vi "Begin.vi"() -> (1 "CameraDevRef":T5)   [LabVIEW 2011]
doc: "Called before other user functions, this VI is expected to open initial I/O refnums, load in file data, and do all program initialization. Notice that the <B>error out</B> terminal is simply used for data flow. Wiring it to other structures or subVIs ensures that this VI runs first."
uses:
  <vilib>/Rock Robotics/WPI/Camera/WPI_CameraDevRef.ctl
  <vilib>/Rock Robotics/WPI/Encoder/WPI_EncoderDevRef.ctl
  <vilib>/Rock Robotics/SystemInterfaces/Encoder/FPGA_EncoderIdx.ctl
  <vilib>/Rock Robotics/SystemInterfaces/Counter/FPGA_CounterCtrSystemIndex.ctl
  <vilib>/Rock Robotics/WPI/Encoder/WPI_EncoderType.ctl
  <vilib>/Rock Robotics/WPI/Joystick/WPI_JoystickDeviceEnum.ctl
  <vilib>/Rock Robotics/SystemInterfaces/DIO/FPGA_DIOPWMChannel.ctl
  <vilib>/Rock Robotics/SystemInterfaces/Typedef/FPGA_TypedefDigitalModule.ctl
  <vilib>/Rock Robotics/WPI/MotorControl/WPI_MotorControlOpen Victor.vi
  Robot Global Data.vi
  <vilib>/Rock Robotics/SystemInterfaces/DIO/FPGA_DIORelayChannel.ctl
  <vilib>/Rock Robotics/WPI/Relay/WPI_RelayDirection.ctl
  <vilib>/Rock Robotics/SystemInterfaces/AI/FPGA_AIChannel.ctl
  <vilib>/Rock Robotics/WPI/Counter/WPI_CounterDigitalInputToDigitalSource.vi
  <vilib>/Rock Robotics/SystemInterfaces/DIO/FPGA_DIOChannel.ctl
  <vilib>/Rock Robotics/SystemInterfaces/AI/FPGA_AIGyroChannel.ctl
  <vilib>/Rock Robotics/WPI/MotorControl/WPI_MotorControlOpen Jaguar.vi
  <vilib>/Rock Robotics/SystemInterfaces/Typedef/FPGA_TypedefAnalogModule.ctl
  <vilib>/Utility/file.llb/Read From Spreadsheet File (DBL).vi
panel:
  out "source":string
  out "code":i32
  out "LDriveEncoder 3":cluster{"status":bool}
  out "EncoderDevRef 3":T1={"DevStatus"={"status"=FALSE, "code"=0, "source"=""}, "EncoderIndex"=enum."Invalid", "CounterIndex"=enum."Invalid", "DistancePerCount"=1.0, "Decoding Type"=enum."4x"}
  out "EncoderDevRef 2":T1={"DevStatus"={"status"=FALSE, "code"=0, "source"=""}, "EncoderIndex"=enum."Invalid", "CounterIndex"=enum."Invalid", "DistancePerCount"=1.0, "Decoding Type"=enum."4x"}
  out "LDriveEncoder 2":errorcluster
  out "EncoderDevRef":T1={"DevStatus"={"status"=FALSE, "code"=0, "source"=""}, "EncoderIndex"=enum."Invalid", "CounterIndex"=enum."Invalid", "DistancePerCount"=1.0, "Decoding Type"=enum."4x"}
  out "LDriveEncoder":errorcluster
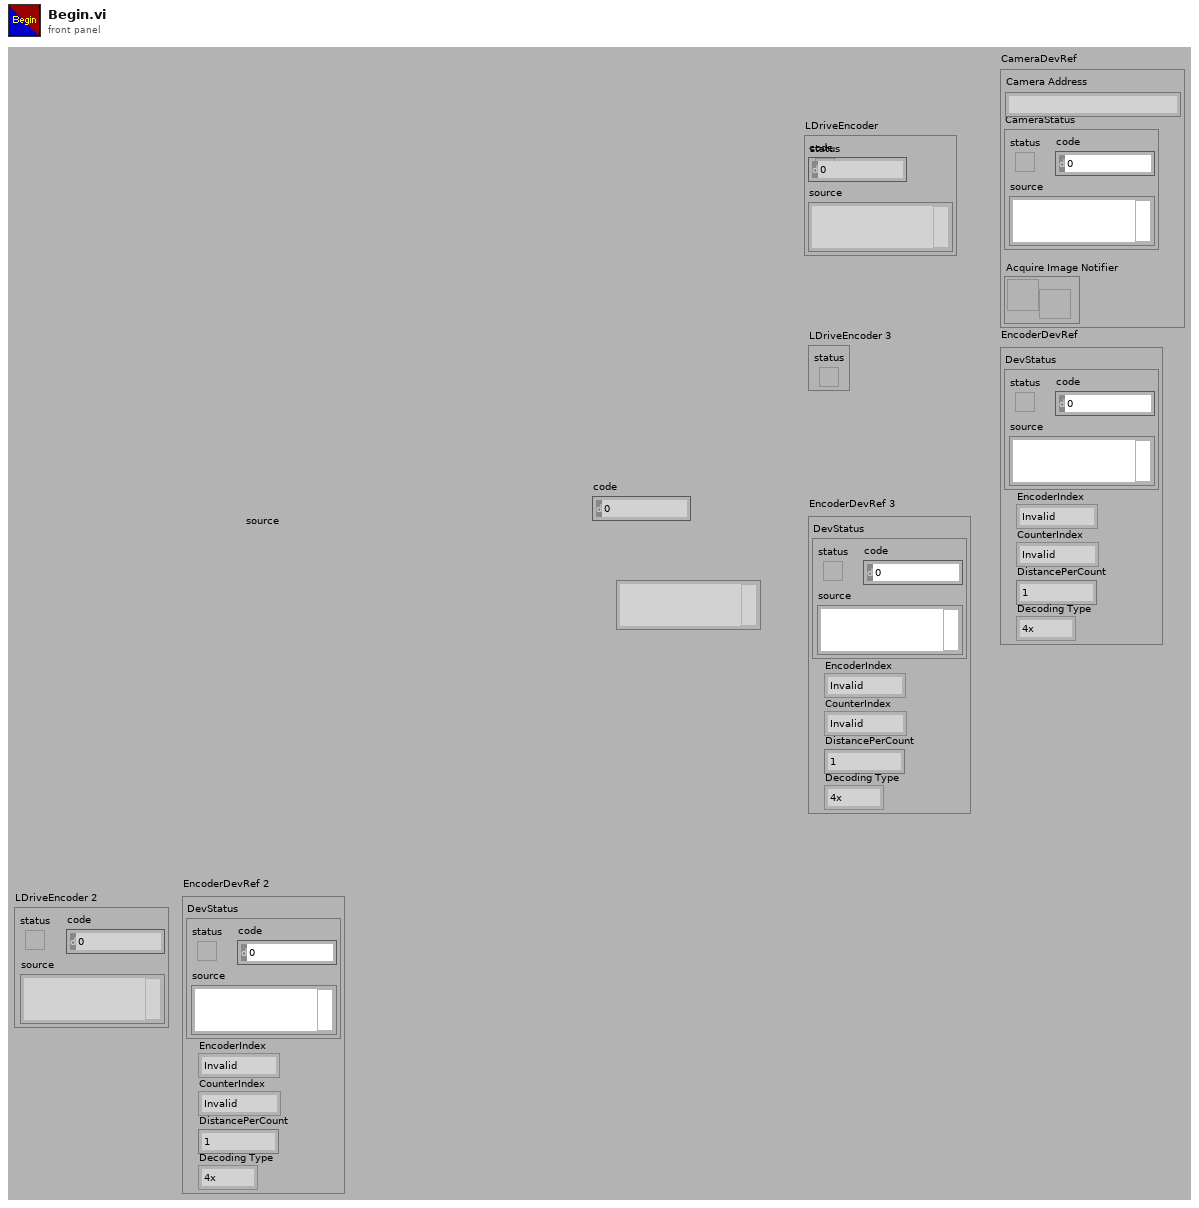
[diagram p1: front panel]
types:
  T1 = typedef "WPI_EncoderDevRef.ctl" = cluster{"DevStatus":errorcluster, "EncoderIndex":T2, "CounterIndex":T3, "DistancePerCount":dbl, "Decoding Type":T4}
  T2 = typedef "FPGA_EncoderIdx.ctl" = enum8{"Enc 0", "Enc 1", "Enc 2", "Enc 3", "Invalid"}
  T3 = typedef "FPGA_CounterCtrSystemIndex.ctl" = enum8{"Ctr 0", "Ctr 1", "Ctr 2", "Ctr 3", "Ctr 4", "Ctr 5", "Ctr 6", "Ctr 7", "Invalid"}
  T4 = typedef "WPI_EncoderType.ctl" = enum16{"1x", "2x", "4x"}
  T5 = typedef "WPI_CameraDevRef.ctl" = cluster{"Camera Address":string, "CameraStatus":errorcluster, "Acquire Image Notifier":refnum<notifier>}
  T6 = typedef "FPGA_TypedefDigitalModule.ctl" = enum16{"Digital Module 1", "Digital Module 2"}
  T7 = typedef "FPGA_DIOPWMChannel.ctl" = enum8{"PWM 1", "PWM 2", "PWM 3", "PWM 4", "PWM 5", "PWM 6", "PWM 7", "PWM 8", "PWM 9", "PWM 10", "Invalid"}
  T8 = typedef "WPI_JoystickDeviceEnum.ctl" = enum16{"USB 1", "USB 2", "USB 3", "USB 4", "Kinect 1", "Kinect 2"}
  T9 = typedef "FPGA_DIORelayChannel.ctl" = enum8{"Relay 1", "Relay 2", "Relay 3", "Relay 4", "Relay 5", "Relay 6", "Relay 7", "Relay 8", "Invalid"}
  T10 = typedef "FPGA_DIOChannel.ctl" = enum8{"DIO 1", "DIO 2", "DIO 3", "DIO 4", "DIO 5", "DIO 6", "DIO 7", "DIO 8", "DIO 9", "DIO 10", "DIO 11", "DIO 12", "DIO 13", "DIO 14", "Invalid"}
  T11 = typedef "WPI_MotorControlDeviceRef.ctl" = cluster{"DeviceStatus":errorcluster, "Type":enum16{"PWM", "CAN"}, "PWM":cluster{"Digital Module":T6, "PWM Channel":T7, "DeadBand":T12}, "CAN":cluster{"Device Number":u8, "Control Mode":T13, "Semaphore":T14, "Max Vout":dbl}, "Invert":bool, "TransformRef":T15, "InvTransformRef":T15}
  T12 = typedef "WPI_PWMDeadband.ctl" = cluster{"Name":string, "maxPositivePwm":i32, "minPositivePwm":i32, "centerPwm":i32, "maxNegativePwm":i32, "minNegativePwm":i32, "angularRange":u16}
  T13 = typedef "WPI_CANJaguar_ControlMode.ctl" = enum8{"Percent VBus", "Current", "Speed", "Position", "Voltage"}
  T14 = typedef "Semaphore RefNum" = refnum<k1>
  T15 = typedef "WPI_PWMTransform_ConPane.ctl" = refnum<vi>
  T16 = typedef "WPI_DigitalInputDevRef.ctl" = cluster{"DevStatus":errorcluster, "DIO Channel":T10, "Digital Module":T6}
  T17 = typedef "FPGA_CounterEncoderSourceConvertionLVSourceType.ctl" = cluster{"DevStatus":errorcluster, "AnalogTriggerMode?":bool, "DigitalMode":cluster{"Digital Module":T6, "DIO Channel":T18}, "AnalogTriggerMode":cluster{"AnalogTriggerIndex":T19, "OutputType":T20}}
  T18 = typedef "FPGA_DIODigitalSourceChannel.ctl" = enum8{"DIO 1", "DIO 2", "DIO 3", "DIO 4", "DIO 5", "DIO 6", "DIO 7", "DIO 8", "DIO 9", "DIO 10", "DIO 11", "DIO 12", "DIO 13", "DIO 14", "Disabled"}
  T19 = typedef "FPGA_AnalogTriggerIndex.ctl" = enum8{"Trig 0", "Trig 1", "Trig 2", "Trig 3", "Trig 4", "Trig 5", "Trig 6", "Trig 7", "Invalid"}
  T20 = typedef "FPGA_AnalogTriggerOutType.ctl" = enum16{"InWindow", "TriggerState", "Rising", "Falling"}
  T21 = typedef "WPI_RelayDevRef.ctl" = cluster{"DevStatus":errorcluster, "Relay Channel":T9, "Digital Module":T6, "Relay Direction":T22}
  T22 = typedef "WPI_RelayDirection.ctl" = enum16{"Both directions", "Forward only", "Reverse only"}
  T23 = typedef "FPGA_AIChannel.ctl" = enum8{"AI 1", "AI 2", "AI 3", "AI 4", "AI 5", "AI 6", "AI 7", "AI 8", "Invalid"}
  T24 = typedef "WPI_JoystickDevRef.ctl" = cluster{"Device":T8}
  T25 = typedef "WPI_AnalogChannelDevRef.ctl" = cluster{"DevStatus":errorcluster, "Analog Module":T26, "Analog Channel":T23}
  T26 = typedef "FPGA_TypedefAnalogModule.ctl" = enum16{"Analog Module 1", "Analog Module 2"}
  T27 = typedef "WPI_CameraImageSize.ctl" = enum16{"640x480", "320x240", "160x120"}
  T28 = cluster{"fps":i32, "compression":i32, "Image Size":T27}
  T29 = typedef "WPI_CameraWhite Balance Values.ctl" = enum16{"Auto", "Fixed indoor", "Fixed outdoor 1", "Fixed outdoor 2", "Fixed fluorescent 1", "Fixed fluorescent 2", "Hold current"}
  T30 = typedef "WPI_CameraExposure Values.ctl" = enum16{"Auto", "Flicker-free 50 Hz", "Flicker-free 60 Hz", "Hold current"}
  T31 = typedef "WPI_ServoDeviceRef.ctl" = cluster{"DeviceStatus":errorcluster, "Digital Module":T6, "PWM Channel":T7, "DeadBand":T12}
  T32 = typedef "FPGA_AIGyroChannel.ctl" = enum8{"AI 1", "AI 2", "Invalid"}
  T33 = typedef "WPI_GyroDevRef.ctl" = cluster{"DevStatus":errorcluster, "Analog Module":T26, "Analog Channel":T23, "Offset":dbl, "Gain (VoltsPerDegree/Second)":dbl}
  T34 = typedef "WPI_UltrasonicDeviceRef.ctl" = cluster{"DevStatus":errorcluster, "Ping Digital Module":T6, "Echo Digital Module":T6, "Ping Channel":T10, "Echo Channel":T10, "CntIndex":T3}
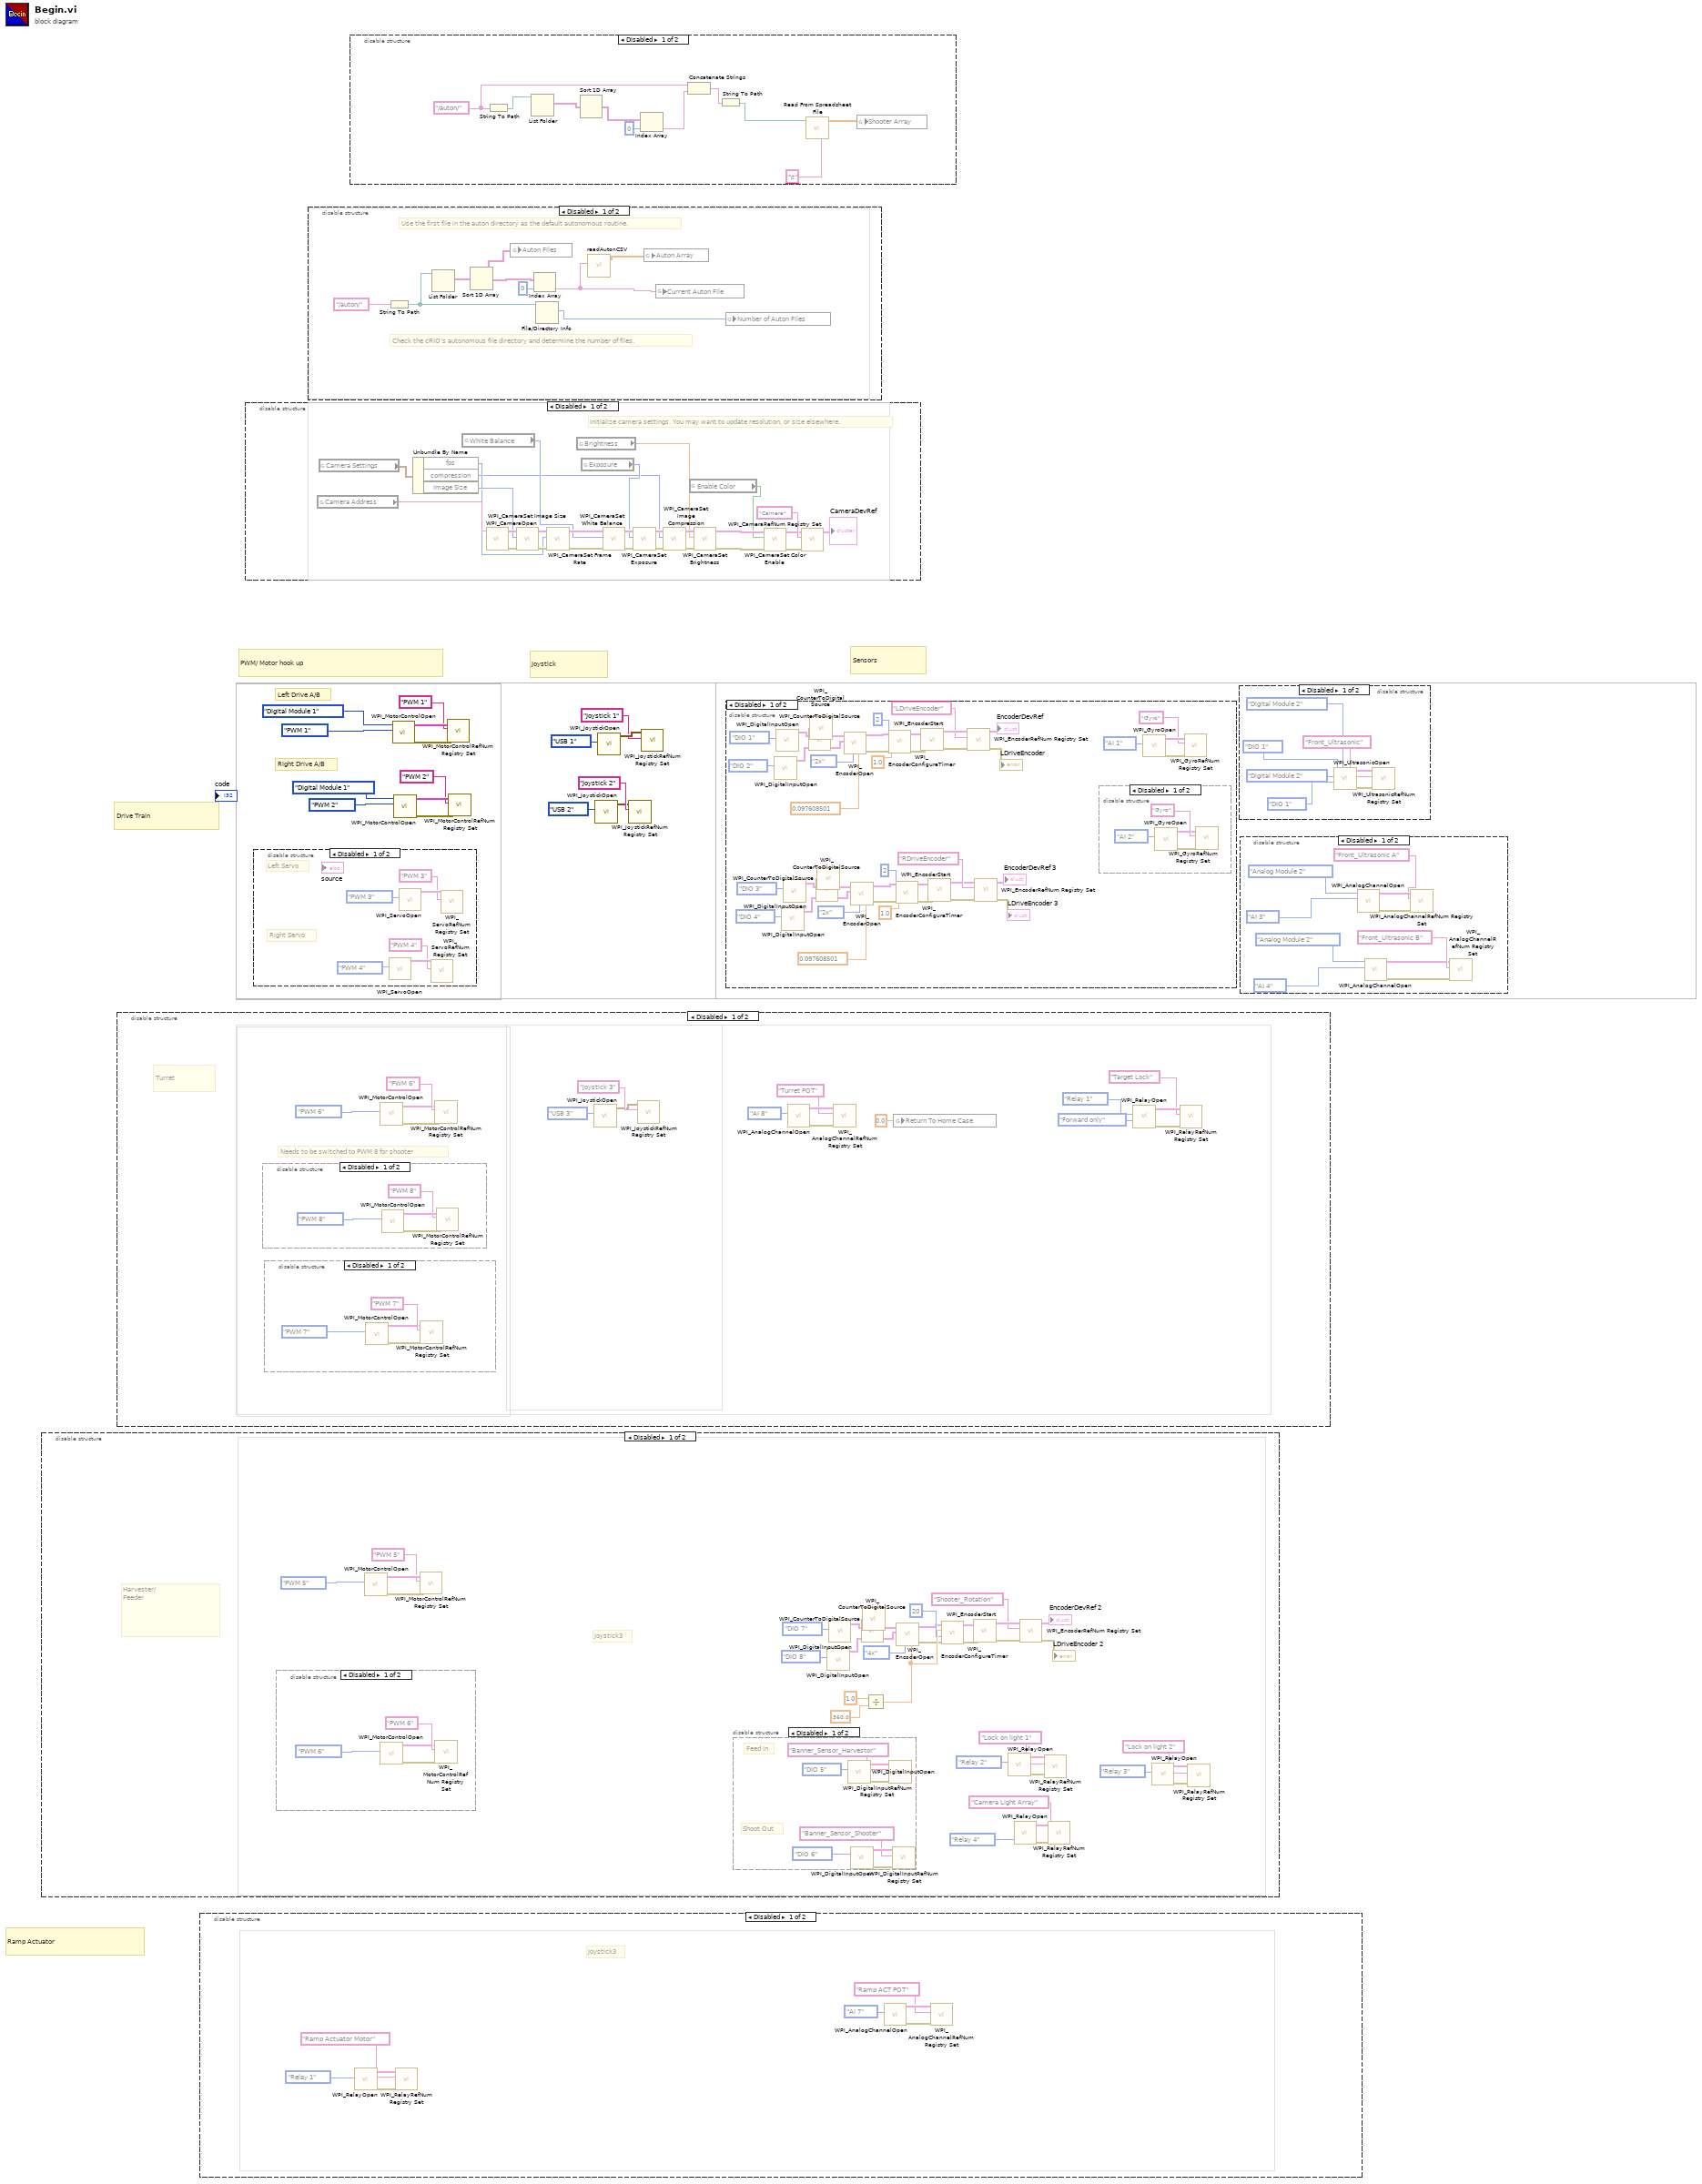
[diagram p0: block diagram]
diagram:
  # "Right Drive A/B"
  # "Left Drive A/B"
  # "Ramp Actuator"
  # "Drive Train"
  # "Sensors"
  # "Joystick"
  # "PWM/ Motor hook up"
  n1 = disable-structure shown="Disabled" {
    frame Disabled {
      # "Harvester/\nFeeder"
      # "Joystick3"
      n2 = disable-structure shown="Disabled" {
        frame Disabled {
          n3 = call-poly <vilib>:"WPI_MotorControlOpen.vi"("PWM Channel"=FPGA_DIOPWMChannel."PWM 6") -> ("error out"=w64:errorcluster, "MotorControlDeviceRef"=w62:T11)  [unwired: 9 in]
          n4 = call <vilib>:"WPI_MotorControlRefNum Registry Set.vi"("error in (no error)"=w64, "refnum name"="PWM 6", "MotorControlDevRef"=w62) -> ()  [unwired: 7 in, 2 out]
        }
        frame Enabled {
        }
      }
      n5 = call-poly <vilib>:"WPI_MotorControlOpen.vi"("PWM Channel"=FPGA_DIOPWMChannel."PWM 5") -> ("error out"=w49:errorcluster, "MotorControlDeviceRef"=w51:T11)  [unwired: 9 in]
      n6 = call <vilib>:"WPI_MotorControlRefNum Registry Set.vi"("error in (no error)"=w49, "refnum name"="PWM 5", "MotorControlDevRef"=w51) -> ()  [unwired: 7 in, 2 out]
      n7 = disable-structure shown="Disabled" {
        frame Disabled {
          # "Shoot Out"
          # "Feed in"
          n8 = call <vilib>:"WPI_DigitalInputOpen.vi"("DIO Channel"=FPGA_DIOChannel."DIO 5") -> ("error out"=w58:errorcluster, "DigitalInputDevRef"=w57:T16)  [unwired: 9 in]
          n9 = call <vilib>:"WPI_DigitalInputOpen.vi"("DIO Channel"=FPGA_DIOChannel."DIO 6") -> ("error out"=w55:errorcluster, "DigitalInputDevRef"=w54:T16)  [unwired: 9 in]
          n10 = call <vilib>:"WPI_DigitalInputRefNum Registry Set.vi"("error in (no error)"=w58, "refnum name"="Banner_Sensor_Harvestor", "DigitalInputDevRef"=w57) -> ()  [unwired: 7 in, 2 out]
          n11 = call <vilib>:"WPI_DigitalInputRefNum Registry Set.vi"("error in (no error)"=w55, "refnum name"="Banner_Sensor_Shooter", "DigitalInputDevRef"=w54) -> ()  [unwired: 7 in, 2 out]
        }
        frame Enabled {
        }
      }
      n12 = call <vilib>:"WPI_DigitalInputOpen.vi"("DIO Channel"=FPGA_DIOChannel."DIO 8") -> ("DigitalInputDevRef"=w33:T16)  [unwired: 9 in, 1 out]
      n13 = call <vilib>:"WPI_DigitalInputOpen.vi"("DIO Channel"=FPGA_DIOChannel."DIO 7") -> ("DigitalInputDevRef"=w30:T16)  [unwired: 9 in, 1 out]
      n14 = call-poly <vilib>:"WPI_CounterToDigitalSource.vi"("DigitalInputDevRef"=w33) -> ("Digital Source"=w34:T17)  [unwired: 6 in]
      n15 = call-poly <vilib>:"WPI_CounterToDigitalSource.vi"("DigitalInputDevRef"=w30) -> ("Digital Source"=w29:T17)  [unwired: 6 in]
      n16 = Divide(x=1.0, y=360.0) -> (x/y=w48:dbl)
      n17 = call <vilib>:"WPI_EncoderOpen.vi"("DistancePerCount"=w48, "Decoding Type"=WPI_EncoderType."4x", "BSource"=w34, "ASource"=w29) -> ("error out"=w37:errorcluster, "EncoderDevRef"=w38:T1)  [unwired: 6 in]
      n18 = call <vilib>:"WPI_EncoderConfigureTimer.vi"("error in (no error)"=w37, "Number Samples to Average"=u8 20, "Minimum Rate"=w48, "EncoderDevRef"=w38) -> ("error out"=w41:errorcluster, "EncoderDevRef"=w40:T1)  [unwired: 6 in]
      n19 = call <vilib>:"WPI_EncoderStart.vi"("error in (no error)"=w41, "EncoderDevRef"=w40) -> ("error out"=w43:errorcluster, "EncoderDevRef"=w42:T1)  [unwired: 8 in]
      n20 = call <vilib>:"WPI_RelayOpen.vi"("Relay Channel"=FPGA_DIORelayChannel."Relay 2") -> ("error out"=w26:errorcluster, "RelayDevRef"=w25:T21)  [unwired: 9 in]
      n21 = call <vilib>:"WPI_RelayOpen.vi"("Relay Channel"=FPGA_DIORelayChannel."Relay 4") -> ("error out"=w28:errorcluster, "RelayDevRef"=w27:T21)  [unwired: 9 in]
      n22 = call <vilib>:"WPI_EncoderRefNum Registry Set.vi"("error in (no error)"=w43, "refnum name"="Shooter_Rotation", "EncoderDevRef"=w42) -> ("error out"=→"LDriveEncoder 2":errorcluster, "EncoderDevRef"=→"EncoderDevRef 2":T1)  [unwired: 7 in]
      n23 = call <vilib>:"WPI_RelayRefNum Registry Set.vi"("error in (no error)"=w26, "refnum name"="Lock on light 1", "RelayDevRef"=w25) -> ()  [unwired: 7 in, 2 out]
      n24 = call <vilib>:"WPI_RelayRefNum Registry Set.vi"("error in (no error)"=w28, "refnum name"="Camera Light Array", "RelayDevRef"=w27) -> ()  [unwired: 7 in, 2 out]
      n25 = call <vilib>:"WPI_RelayOpen.vi"("Relay Channel"=FPGA_DIORelayChannel."Relay 3") -> ("error out"=w17:errorcluster, "RelayDevRef"=w18:T21)  [unwired: 9 in]
      n26 = call <vilib>:"WPI_RelayRefNum Registry Set.vi"("error in (no error)"=w17, "refnum name"="Lock on light 2", "RelayDevRef"=w18) -> ()  [unwired: 7 in, 2 out]
    }
    frame Enabled {
    }
  }
  n27 = disable-structure shown="Disabled" {
    frame Disabled {
      # "Needs to be switched to PWM 8 for shooter"
      # "Turret"
      n28 = disable-structure shown="Disabled" {
        frame Disabled {
          n29 = call-poly <vilib>:"WPI_MotorControlOpen.vi"("PWM Channel"=FPGA_DIOPWMChannel."PWM 8") -> ("error out"=w86:errorcluster, "MotorControlDeviceRef"=w88:T11)  [unwired: 9 in]
          n30 = call <vilib>:"WPI_MotorControlRefNum Registry Set.vi"("error in (no error)"=w86, "refnum name"="PWM 8", "MotorControlDevRef"=w88) -> ()  [unwired: 7 in, 2 out]
        }
        frame Enabled {
        }
      }
      n31 = disable-structure shown="Disabled" {
        frame Disabled {
          n32 = call-poly <vilib>:"WPI_MotorControlOpen.vi"("PWM Channel"=FPGA_DIOPWMChannel."PWM 7") -> ("error out"=w85:errorcluster, "MotorControlDeviceRef"=w83:T11)  [unwired: 9 in]
          n33 = call <vilib>:"WPI_MotorControlRefNum Registry Set.vi"("error in (no error)"=w85, "refnum name"="PWM 7", "MotorControlDevRef"=w83) -> ()  [unwired: 7 in, 2 out]
        }
        frame Enabled {
        }
      }
      n34 = call-poly <vilib>:"WPI_MotorControlOpen.vi"("PWM Channel"=FPGA_DIOPWMChannel."PWM 6") -> ("error out"=w81:errorcluster, "MotorControlDeviceRef"=w79:T11)  [unwired: 9 in]
      n35 = call <vilib>:"WPI_MotorControlRefNum Registry Set.vi"("error in (no error)"=w81, "refnum name"="PWM 6", "MotorControlDevRef"=w79) -> ()  [unwired: 7 in, 2 out]
      n36 = call <vilib>:"WPI_JoystickOpen.vi"("JoystickDevice"=WPI_JoystickDeviceEnum."USB 3") -> ("JoystickDevRef"=w76:T24)  [unwired: 10 in]
      n37 = call <vilib>:"WPI_JoystickRefNum Registry Set.vi"("refnum name"="Joystick 3", "JoystickDevRef"=w76) -> ()  [unwired: 8 in, 2 out]
      n38 = call <vilib>:"WPI_AnalogChannelOpen.vi"("Analog Channel"=FPGA_AIChannel."AI 8") -> ("error out"=w68:errorcluster, "AIDeviceRef"=w69:T25)  [unwired: 9 in]
      n39 = call <vilib>:"WPI_AnalogChannelRefNum Registry Set.vi"("error in (no error)"=w68, "refnum name"="Turret POT", "AIDeviceRef"=w69) -> ()  [unwired: 7 in, 2 out]
      n40 = global write "Robot Global Data.vi" "Return To Home Case"(0.0 ("Return To Home Case")) -> ()
      n41 = call <vilib>:"WPI_RelayOpen.vi"("Relay Direction"=WPI_RelayDirection."Forward only", "Relay Channel"=FPGA_DIORelayChannel."Relay 1") -> ("error out"=w73:errorcluster, "RelayDevRef"=w74:T21)  [unwired: 8 in]
      n42 = call <vilib>:"WPI_RelayRefNum Registry Set.vi"("error in (no error)"=w73, "refnum name"="Target Lock", "RelayDevRef"=w74) -> ()  [unwired: 7 in, 2 out]
    }
    frame Enabled {
    }
  }
  n43 = disable-structure shown="Disabled" {
    frame Disabled {
      # "Joystick3"
      n44 = call <vilib>:"WPI_RelayOpen.vi"("Relay Channel"=FPGA_DIORelayChannel."Relay 1") -> ("error out"=w93:errorcluster, "RelayDevRef"=w92:T21)  [unwired: 9 in]
      n45 = call <vilib>:"WPI_RelayRefNum Registry Set.vi"("error in (no error)"=w93, "refnum name"="Ramp Actuator Motor", "RelayDevRef"=w92) -> ()  [unwired: 7 in, 2 out]
      n46 = call <vilib>:"WPI_AnalogChannelOpen.vi"("Analog Channel"=FPGA_AIChannel."AI 7") -> ("error out"=w96:errorcluster, "AIDeviceRef"=w97:T25)  [unwired: 9 in]
      n47 = call <vilib>:"WPI_AnalogChannelRefNum Registry Set.vi"("error in (no error)"=w96, "refnum name"="Ramp ACT POT", "AIDeviceRef"=w97) -> ()  [unwired: 7 in, 2 out]
    }
    frame Enabled {
    }
  }
  n48 = disable-structure shown="Disabled" {
    frame Disabled {
      # "Initialize camera settings. You may want to update resolution, or size elsewhere."
      n49 = global read "Robot Global Data.vi" "Camera Address"() -> (w111:string)
      n50 = global read "Robot Global Data.vi" "Camera Settings"() -> (w110:T28)
      n51 = Unbundle By Name(w110) -> ("fps"=w108:i32, "compression"=w105:i32, "Image Size"=w109:T27)
      n52 = global read "Robot Global Data.vi" "White Balance"() -> (w107:T29)
      n53 = call <vilib>:"WPI_CameraOpen.vi"("Camera Address"=w111) -> ("error out"=w117:errorcluster, "CameraDevRef"=w118:T5)  [unwired: 1 in, 8 out]
      n54 = call <vilib>:"WPI_CameraSet Image Size.vi"("error in (no error)"=w117, "Image Size"=w109, "CameraDevRef"=w118) -> ("error out"=w116:errorcluster, "CameraDevRef Out"=w119:T5)  [unwired: 7 out]
      n55 = call <vilib>:"WPI_CameraSet Frame Rate.vi"("error in (no error)"=w116, "Frame Rate (fps)"=w108, "CameraDevRef"=w119) -> ("error out"=w115:errorcluster, "CameraDevRef Out"=w121:T5)  [unwired: 7 out]
      n56 = global read "Robot Global Data.vi" "Brightness"() -> (w104:dbl)
      n57 = global read "Robot Global Data.vi" "Exposure"() -> (w106:T30)
      n58 = call <vilib>:"WPI_CameraSet White Balance.vi"("error in (no error)"=w115, "White Balance"=w107, "CameraDevRef"=w121) -> ("error out"=w114:errorcluster, "CameraDevRef Out"=w120:T5)  [unwired: 7 out]
      n59 = call <vilib>:"WPI_CameraSet Exposure.vi"("error in (no error)"=w114, "Exposure"=w106, "CameraDevRef"=w120) -> ("error out"=w113:errorcluster, "CameraDevRef Out"=w123:T5)  [unwired: 7 out]
      n60 = call <vilib>:"WPI_CameraSet Image Compression.vi"("error in (no error)"=w113, "Compression"=w105, "CameraDevRef"=w123) -> ("error out"=w112:errorcluster, "CameraDevRef Out"=w122:T5)  [unwired: 7 out]
      n61 = global read "Robot Global Data.vi" "Enable Color"() -> (w99:bool)
      n62 = call <vilib>:"WPI_CameraSet Brightness.vi"("error in (no error)"=w112, "Brightness"=w104, "CameraDevRef"=w122) -> ("error out"=w102:errorcluster, "CameraDevRef Out"=w103:T5)  [unwired: 7 out]
      n63 = call <vilib>:"WPI_CameraSet Color Enable.vi"("error in (no error)"=w102, "Color Enabled"=w99, "CameraDevRef"=w103) -> ("error out"=w100:errorcluster, "CameraDevRef Out"=w101:T5)  [unwired: 7 in]
      n64 = call <vilib>:"WPI_CameraRefNum Registry Set.vi"("error in (no error)"=w100, "refnum name"="Camera", "CameraDevRef"=w101) -> ("CameraDevRef"=→"CameraDevRef":T5)  [unwired: 8 out]
    }
    frame Enabled {
    }
  }
  n65 = disable-structure shown="Disabled" {
    frame Disabled {
      # "Right Servo"
      # "Left Servo"
      n66 = call <vilib>:"WPI_ServoOpen.vi"("PWM Channel"=FPGA_DIOPWMChannel."PWM 4") -> ("ServoDeviceRef"=w127:T31)  [unwired: 9 in, 1 out]
      n67 = call <vilib>:"WPI_ServoOpen.vi"("PWM Channel"=FPGA_DIOPWMChannel."PWM 3") -> ("ServoDeviceRef"=w129:T31)  [unwired: 9 in, 1 out]
      n68 = call <vilib>:"WPI_ServoRefNum Registry Set.vi"("refnum name"="PWM 4", "ServoDeviceRef"=w127) -> ()  [unwired: 8 in, 2 out]
      n69 = call <vilib>:"WPI_ServoRefNum Registry Set.vi"("refnum name"="PWM 3", "ServoDeviceRef"=w129) -> ()  [unwired: 8 in, 2 out]
    }
    frame Enabled {
    }
  }
  n70 = disable-structure shown="Disabled" {
    frame Disabled {
      # "Check the cRIO's autonomous file directory and determine the number of files."
      # "Use the first file in the auton directory as the default autonomous routine."
      n71 = String To Path(string="/auton/") -> (path=w137:path)
      n72 = List Folder(path=w137) -> (filenames=w136:string[])  [unwired: 1 in, 5 out]
      n73 = Sort 1D Array(array=w136) -> (sorted array=w131:string[])
      n74 = global write "Robot Global Data.vi" "Auton Files"(w131) -> ()
      n75 = Index Array(array=w131, index=0) -> (element=w133:string)
      n76 = File/Directory Info(path=w137) -> (size=w134:i64)  [unwired: 1 in, 6 out]
      n77 = call "readAutonCSV.vi"("AutonFile"=w133) -> ("AutonArray"=w132:dbl[][])  [unwired: 7 in]
      n78 = global write "Robot Global Data.vi" "Auton Array"(w132) -> ()
      n79 = global write "Robot Global Data.vi" "Current Auton File"(w133) -> ()
      n80 = global write "Robot Global Data.vi" "Number of Auton Files"(w134) -> ()
    }
    frame Enabled {
    }
  }
  n81 = disable-structure shown="Disabled" {
    frame Disabled {
      w147 = "/auton/" ("string")
      n82 = String To Path(string=w147) -> (path=w148:path)
      n83 = List Folder(path=w148) -> (filenames=w146:string[])  [unwired: 1 in, 5 out]
      n84 = Sort 1D Array(array=w146) -> (sorted array=w145:string[])
      n85 = Index Array(array=w145, index=0) -> (element=w143:string)
      n86 = Concatenate Strings(w147, w143) -> (w142:string)
      n87 = String To Path(string=w142) -> (path=w141:path)
      n88 = call-poly <vilib>:"Read From Spreadsheet File.vi"("delimiter (\\t)"="\t" ("delimiter (\\t)"), "file path (dialog if empty)"=w141) -> ("all rows"=w139:dbl[][])  [unwired: 5 in, 4 out]
      n89 = global write "Robot Global Data.vi" "Shooter Array"(w139) -> ()
    }
    frame Enabled {
    }
  }
  n90 = call-poly <vilib>:"WPI_MotorControlOpen.vi"("PWM Channel"=FPGA_DIOPWMChannel."PWM 1", "Digital Module (Module 1)"=FPGA_TypedefDigitalModule."Digital Module 1") -> ("error out"=w3:errorcluster, "MotorControlDeviceRef"=w6:T11)  [unwired: 8 in]
  n91 = call-poly <vilib>:"WPI_MotorControlOpen.vi"("PWM Channel"=FPGA_DIOPWMChannel."PWM 2", "Digital Module (Module 1)"=FPGA_TypedefDigitalModule."Digital Module 1") -> ("error out"=w4:errorcluster, "MotorControlDeviceRef"=w9:T11)  [unwired: 8 in]
  n92 = call <vilib>:"WPI_MotorControlRefNum Registry Set.vi"("error in (no error)"=w3, "refnum name"="PWM 1", "MotorControlDevRef"=w6) -> ()  [unwired: 7 in, 2 out]
  n93 = call <vilib>:"WPI_MotorControlRefNum Registry Set.vi"("error in (no error)"=w4, "refnum name"="PWM 2", "MotorControlDevRef"=w9) -> ()  [unwired: 7 in, 2 out]
  n94 = call <vilib>:"WPI_JoystickOpen.vi"("JoystickDevice"=WPI_JoystickDeviceEnum."USB 2") -> ("JoystickDevRef"=w13:T24)  [unwired: 10 in]
  n95 = call <vilib>:"WPI_JoystickOpen.vi"("JoystickDevice"=WPI_JoystickDeviceEnum."USB 1") -> ("JoystickDevRef"=w16:T24)  [unwired: 10 in]
  n96 = call <vilib>:"WPI_JoystickRefNum Registry Set.vi"("refnum name"="Joystick 2", "JoystickDevRef"=w13) -> ()  [unwired: 8 in, 2 out]
  n97 = call <vilib>:"WPI_JoystickRefNum Registry Set.vi"("refnum name"="Joystick 1", "JoystickDevRef"=w16) -> ()  [unwired: 8 in, 2 out]
  n98 = disable-structure shown="Disabled" {
    frame Disabled {
      n99 = call <vilib>:"WPI_DigitalInputOpen.vi"("DIO Channel"=FPGA_DIOChannel."DIO 2") -> ("DigitalInputDevRef"=w172:T16)  [unwired: 9 in, 1 out]
      n100 = call <vilib>:"WPI_DigitalInputOpen.vi"("DIO Channel"=FPGA_DIOChannel."DIO 1") -> ("DigitalInputDevRef"=w169:T16)  [unwired: 9 in, 1 out]
      n101 = call <vilib>:"WPI_DigitalInputOpen.vi"("DIO Channel"=FPGA_DIOChannel."DIO 4") -> ("DigitalInputDevRef"=w163:T16)  [unwired: 9 in, 1 out]
      n102 = call <vilib>:"WPI_DigitalInputOpen.vi"("DIO Channel"=FPGA_DIOChannel."DIO 3") -> ("DigitalInputDevRef"=w166:T16)  [unwired: 9 in, 1 out]
      n103 = call-poly <vilib>:"WPI_CounterToDigitalSource.vi"("DigitalInputDevRef"=w172) -> ("Digital Source"=w173:T17)  [unwired: 6 in]
      n104 = call-poly <vilib>:"WPI_CounterToDigitalSource.vi"("DigitalInputDevRef"=w169) -> ("Digital Source"=w168:T17)  [unwired: 6 in]
      n105 = call-poly <vilib>:"WPI_CounterToDigitalSource.vi"("DigitalInputDevRef"=w163) -> ("Digital Source"=w162:T17)  [unwired: 6 in]
      n106 = call-poly <vilib>:"WPI_CounterToDigitalSource.vi"("DigitalInputDevRef"=w166) -> ("Digital Source"=w167:T17)  [unwired: 6 in]
      n107 = call <vilib>:"WPI_EncoderOpen.vi"("DistancePerCount"=0.097608501, "Decoding Type"=WPI_EncoderType."2x", "BSource"=w173, "ASource"=w168) -> ("error out"=w177:errorcluster, "EncoderDevRef"=w178:T1)  [unwired: 6 in]
      n108 = call <vilib>:"WPI_EncoderOpen.vi"("DistancePerCount"=0.097608501, "Decoding Type"=WPI_EncoderType."2x", "BSource"=w162, "ASource"=w167) -> ("error out"=w158:errorcluster, "EncoderDevRef"=w157:T1)  [unwired: 6 in]
      n109 = call <vilib>:"WPI_EncoderConfigureTimer.vi"("error in (no error)"=w177, "Number Samples to Average"=u8 2, "Minimum Rate"=1.0, "EncoderDevRef"=w178) -> ("error out"=w182:errorcluster, "EncoderDevRef"=w181:T1)  [unwired: 6 in]
      n110 = call <vilib>:"WPI_EncoderConfigureTimer.vi"("error in (no error)"=w158, "Number Samples to Average"=u8 2, "Minimum Rate"=1.0, "EncoderDevRef"=w157) -> ("error out"=w153:errorcluster, "EncoderDevRef"=w154:T1)  [unwired: 6 in]
      n111 = call <vilib>:"WPI_EncoderStart.vi"("error in (no error)"=w182, "EncoderDevRef"=w181) -> ("error out"=w184:errorcluster, "EncoderDevRef"=w183:T1)  [unwired: 8 in]
      n112 = call <vilib>:"WPI_EncoderStart.vi"("error in (no error)"=w153, "EncoderDevRef"=w154) -> ("error out"=w151:errorcluster, "EncoderDevRef"=w152:T1)  [unwired: 8 in]
      n113 = call <vilib>:"WPI_EncoderRefNum Registry Set.vi"("error in (no error)"=w184, "refnum name"="LDriveEncoder", "EncoderDevRef"=w183) -> ("error out"=→"LDriveEncoder":errorcluster, "EncoderDevRef"=→"EncoderDevRef":T1)  [unwired: 7 in]
      n114 = call <vilib>:"WPI_EncoderRefNum Registry Set.vi"("error in (no error)"=w151, "refnum name"="RDriveEncoder", "EncoderDevRef"=w152) -> ("error out"=→"LDriveEncoder 3":errorcluster, "EncoderDevRef"=→"EncoderDevRef 3":T1)  [unwired: 7 in]
      n115 = disable-structure shown="Disabled" {
        frame Disabled {
          n116 = call <vilib>:"WPI_GyroOpen.vi"("Analog Channel"=FPGA_AIGyroChannel."AI 2") -> ("error out"=w191:errorcluster, "GyroDevRef"=w192:T33)  [unwired: 8 in, 1 out]
          n117 = call <vilib>:"WPI_GyroRefNum Registry Set.vi"("error in (no error)"=w191, "refnum name"="Gyro", "GyroDevRef"=w192) -> ()  [unwired: 7 in, 2 out]
        }
        frame Enabled {
        }
      }
      n118 = call <vilib>:"WPI_GyroOpen.vi"("Analog Channel"=FPGA_AIGyroChannel."AI 1") -> ("error out"=w190:errorcluster, "GyroDevRef"=w189:T33)  [unwired: 8 in, 1 out]
      n119 = call <vilib>:"WPI_GyroRefNum Registry Set.vi"("error in (no error)"=w190, "refnum name"="Gyro", "GyroDevRef"=w189) -> ()  [unwired: 7 in, 2 out]
    }
    frame Enabled {
    }
  }
  n120 = disable-structure shown="Disabled" {
    frame Disabled {
      n121 = call <vilib>:"WPI_UltrasonicOpen.vi"("Ping Digital Module (Module 1)"=FPGA_TypedefDigitalModule."Digital Module 2", "Echo DIO Channel"=FPGA_DIOChannel."DIO 1", "Echo Digital Module (Module 1)"=FPGA_TypedefDigitalModule."Digital Module 2", "Ping DIO Channel"=FPGA_DIOChannel."DIO 1") -> ("error out"=w201:errorcluster, "UltrasonicDevRef"=w200:T34)  [unwired: 6 in]
      n122 = call <vilib>:"WPI_UltrasonicRefNum Registry Set.vi"("error in (no error)"=w201, "refnum name"="Front_Ultrasonic", "UltrasonicDevRef"=w200) -> ()  [unwired: 7 in, 2 out]
    }
    frame Enabled {
    }
  }
  n123 = disable-structure shown="Disabled" {
    frame Disabled {
      n124 = call <vilib>:"WPI_AnalogChannelOpen.vi"("Analog Channel"=FPGA_AIChannel."AI 3", "Analog Module (Module 1)"=FPGA_TypedefAnalogModule."Analog Module 2") -> ("error out"=w207:errorcluster, "AIDeviceRef"=w206:T25)  [unwired: 8 in]
      n125 = call <vilib>:"WPI_AnalogChannelOpen.vi"("Analog Channel"=FPGA_AIChannel."AI 4", "Analog Module (Module 1)"=FPGA_TypedefAnalogModule."Analog Module 2") -> ("error out"=w202:errorcluster, "AIDeviceRef"=w203:T25)  [unwired: 8 in]
      n126 = call <vilib>:"WPI_AnalogChannelRefNum Registry Set.vi"("error in (no error)"=w207, "refnum name"="Front_Ultrasonic A", "AIDeviceRef"=w206) -> ()  [unwired: 7 in, 2 out]
      n127 = call <vilib>:"WPI_AnalogChannelRefNum Registry Set.vi"("error in (no error)"=w202, "refnum name"="Front_Ultrasonic B", "AIDeviceRef"=w203) -> ()  [unwired: 7 in, 2 out]
    }
    frame Enabled {
    }
  }
